vi "SliderExpansion.vi"(8 "Error Out":errorcluster, 10 "Slider color":u32(colorbox), 11 "Slide Refnum":refnum<vi>) -> (0 "Error Out":errorcluster)   [LabVIEW 2021]
doc: "Animating slider filling to maximum value in choosen color. Comments in Polish."
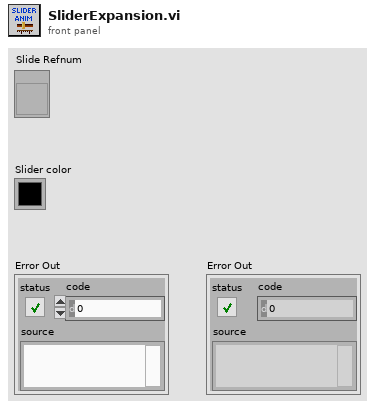
[diagram p1: front panel]
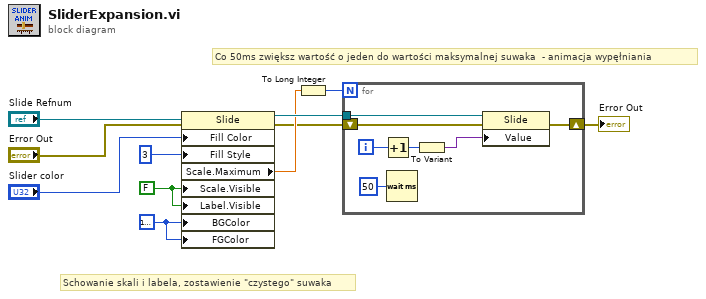
[diagram p0: block diagram]
diagram:
  w3 = u32 16777216
  w1 = FALSE ("Scale.Visible")
  # "Co 50ms zwiększ wartość o jeden do wartości maksymalnej suwaka  - animacja wypęłniania"
  # "Schowanie skali i labela, zostawienie \"czystego\" suwaka"
  n1 = property class="Slide"(reference="Slide Refnum", error in="Error Out", "Fill Color"="Slider color", "Fill Style"=3, "Scale.Visible"=w1, "Label.Visible"=w1, "BGColor"=w3, "FGColor"=w3) -> (reference out=w9:refnum<vi>, error out=w2:errorcluster, "Scale.Maximum"=w7:dbl)
  n2 = To Long Integer(number=w7) -> (32bit integer=w8:i32)
  n3 = for {
    N: w8 -> [_]
    tunnel: w9 -> [w18]
    shift-right: [w16] -> w6
    shift-left: w2 -> [w17]
    i -> [w13]
    n4 = Increment(x=w13) -> (x+1=w12:i32)
    n5 = Wait (ms)(milliseconds to wait=u32 50) -> ()  [unwired: 1 out]
    n6 = To Variant(anything=w12) -> (Variant=w14:variant)
    n7 = property class="Slide"(reference=w18, error in=w17, "Value"=w14) -> (error out=w16:errorcluster)  [unwired: 1 out]
  }
  "Error Out" <- w6
